vi "autonomous hard code.vi"   [LabVIEW 2012]
uses:
  <vilib>/Platform/TimedLoop/XDataNode/timing_clust.ctl
  <vilib>/Platform/TimedLoop/XDataNode/nitl_modes.ctl
  <vilib>/Platform/TimedLoop/XDataNode/wakeup.ctl
  <vilib>/Rock Robotics/WPI/RobotDrive/WPI_RobotDriveArcadeDrive_Standard(NoSaturation).vi
  <vilib>/Rock Robotics/WPI/RobotDrive/WPI_RobotDriveGetSetRefNum.vi
  <vilib>/platform/TimedLoop/XDataNode/XDataNode.xnode
  <vilib>/Platform/TimedLoop/XDataNode/XDNodeRunTimeDep.lvlib
types:
  T1 = typedef "XDNodeRunTimeDep.lvlib/timing_clust.ctl" = cluster{"Expected End [f-1]":u64, "Actual End [f-1]":u64, "Finished Late? [f-1]":bool, "Expected End [i-1]":u64, "Actual End [i-1]":u64, "Finished Late? [i-1]":bool, "Expected Start [i]":u64, "Actual Start [i]":u64, "Expected Start [f]":u64, "Actual Start [f]":u64, "Source Name":string, "Structure Name":string, "Period":i64, "Deadline":i64, "Offset":i64, "Start":i64, "Priority":i32, "Timeout":i32, "Mode":T2, "Wakeup Reason":T3, "Error":errorcluster, "Source Type":string, "Secondary Source Type":string, "Global End Time":u64, "Global Start Time":u64, "Frame Duration":u64, "Iteration Duration":u64, "Assigned CPU":i32, "I/O Scan Engine Mode":u32}
  T2 = typedef "XDNodeRunTimeDep.lvlib/nitl_modes.ctl" = enum32{"No Change", "Process missed periods, maintain original phase", "Discard missed periods, maintain original phase", "Process missed periods, ignore original phase", "Discard missed periods, ignore original phase"}
  T3 = typedef "XDNodeRunTimeDep.lvlib/wakeup.ctl" = enum32{"Normal", "Aborted", "Asynchronous wakeup", "Timing source error", "Timed loop error", "Timeout"}
  T4 = typedef "WPI_RobotDriveDevRef.ctl" = cluster{"DevStatus":errorcluster, "Motors[]":T5[], "Square Inputs":bool, "Max Output":dbl, "Isochronous":bool}
  T5 = typedef "WPI_MotorControlDeviceRef.ctl" = cluster{"DeviceStatus":errorcluster, "Type":enum16{"PWM", "CAN"}, "PWM":cluster{"Digital Module":T6, "PWM Channel":T7, "DeadBand":T8}, "CAN":cluster{"Device Number":u8, "Control Mode":T9, "Semaphore":T10, "Max Vout":dbl}, "Invert":bool, "TransformRef":T11, "InvTransformRef":T11}
  T6 = typedef "FPGA_TypedefDigitalModule.ctl" = enum16{"Digital Module 1", "Digital Module 2"}
  T7 = typedef "FPGA_DIOPWMChannel.ctl" = enum8{"PWM 1", "PWM 2", "PWM 3", "PWM 4", "PWM 5", "PWM 6", "PWM 7", "PWM 8", "PWM 9", "PWM 10", "Invalid"}
  T8 = typedef "WPI_PWMDeadband.ctl" = cluster{"Name":string, "maxPositivePwm":i32, "minPositivePwm":i32, "centerPwm":i32, "maxNegativePwm":i32, "minNegativePwm":i32, "angularRange":u16}
  T9 = typedef "WPI_CANJaguar_ControlMode.ctl" = enum8{"Percent VBus", "Current", "Speed", "Position", "Voltage"}
  T10 = typedef "Semaphore RefNum" = refnum<k1>
  T11 = typedef "WPI_PWMTransform_ConPane.ctl" = refnum<vi>
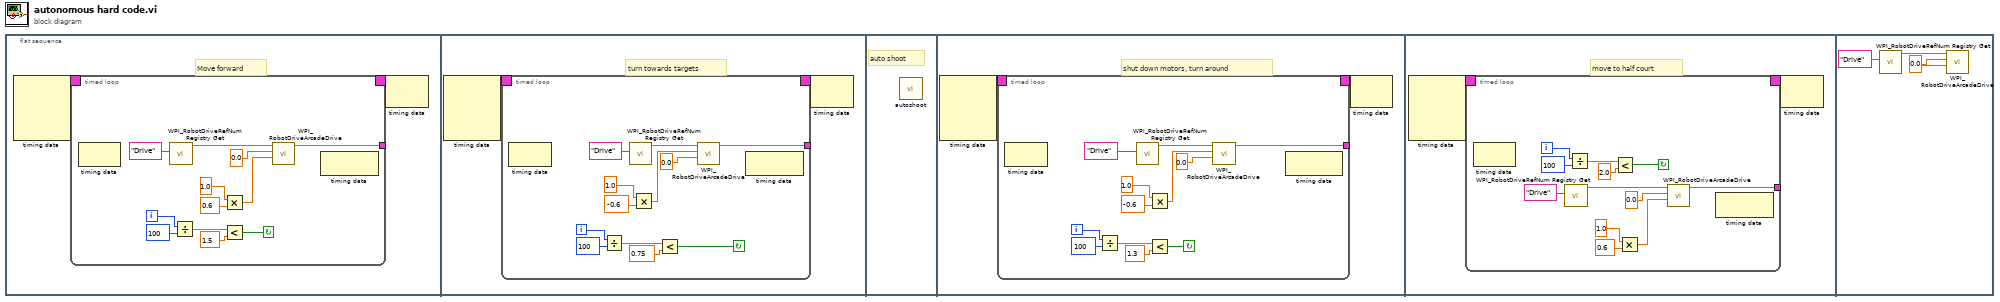
[diagram p0: block diagram]
diagram:
  n1 = flat-sequence {
    frame #0 {
      # "Move forward"
      n2 = node-c288() -> (w2:T1)  [unwired: 4 in]
      n3 = timed-loop {
        timing: w2 -> [_]
        timing-out: [_] -> w1
        tunnel: [w8] -> _
        i -> [w7]
        stop <- w14 continue-if-true
        n4 = node-c288() -> ()  [unwired: 1 in, 1 out]
        n5 = call <vilib>:"WPI_RobotDriveRefNum Registry Get.vi"("refnum name"="Drive") -> ("RobotDriveDevRef"=w10:T4)  [unwired: 9 in, 1 out]
        n6 = Divide(x=w7, y=100) -> (x/y=w12:dbl)
        n7 = Multiply(x=1.0, y=0.6) -> (x*y=w3:dbl)
        n8 = Less?(x=w12, y=1.5) -> (x < y?=w14:bool)
        n9 = call-poly <vilib>:"WPI_RobotDriveArcadeDrive.vi"("Y axis value"=w3, "X axis value"=0.0 ("Y axis value"), "RobotDriveDevRef"=w10) -> ("RobotDriveDevRef"=w8:T4)  [unwired: 6 in, 2 out]
        n10 = node-c288() -> ()  [unwired: 1 in, 1 out]
      }
      n11 = node-c288(w1) -> ()  [unwired: 1 out]
    }
    frame #1 {
      # "turn towards targets"
      n12 = node-c288() -> (w20:T1)  [unwired: 4 in]
      n13 = timed-loop {
        timing: w20 -> [_]
        timing-out: [_] -> w19
        tunnel: [w24] -> _
        i -> [w23]
        stop <- w32 continue-if-true
        n14 = node-c288() -> ()  [unwired: 1 in, 1 out]
        n15 = Divide(x=w23, y=100) -> (x/y=w30:dbl)
        n16 = call <vilib>:"WPI_RobotDriveRefNum Registry Get.vi"("refnum name"="Drive") -> ("RobotDriveDevRef"=w28:T4)  [unwired: 9 in, 1 out]
        n17 = Multiply(x=1.0, y=-0.6) -> (x*y=w27:dbl)
        n18 = Less?(x=w30, y=0.75) -> (x < y?=w32:bool)
        n19 = call-poly <vilib>:"WPI_RobotDriveArcadeDrive.vi"("Y axis value"=0.0, "X axis value"=w27, "RobotDriveDevRef"=w28) -> ("RobotDriveDevRef"=w24:T4)  [unwired: 6 in, 2 out]
        n20 = node-c288() -> ()  [unwired: 1 in, 1 out]
      }
      n21 = node-c288(w19) -> ()  [unwired: 1 out]
    }
    frame #2 {
      # "auto shoot"
      n22 = call "autoshoot.vi"() -> ()  [unwired: 12 in]
    }
    frame #3 {
      # "shut down motors, turn around"
      n23 = node-c288() -> (w38:T1)  [unwired: 4 in]
      n24 = timed-loop {
        timing: w38 -> [_]
        timing-out: [_] -> w37
        tunnel: [w42] -> _
        i -> [w41]
        stop <- w50 continue-if-true
        n25 = node-c288() -> ()  [unwired: 1 in, 1 out]
        n26 = Divide(x=w41, y=100) -> (x/y=w48:dbl)
        n27 = call <vilib>:"WPI_RobotDriveRefNum Registry Get.vi"("refnum name"="Drive") -> ("RobotDriveDevRef"=w46:T4)  [unwired: 9 in, 1 out]
        n28 = Multiply(x=1.0, y=-0.6) -> (x*y=w45:dbl)
        n29 = Less?(x=w48, y=1.3) -> (x < y?=w50:bool)
        n30 = call-poly <vilib>:"WPI_RobotDriveArcadeDrive.vi"("Y axis value"=0.0, "X axis value"=w45, "RobotDriveDevRef"=w46) -> ("RobotDriveDevRef"=w42:T4)  [unwired: 6 in, 2 out]
        n31 = node-c288() -> ()  [unwired: 1 in, 1 out]
      }
      n32 = node-c288(w37) -> ()  [unwired: 1 out]
    }
    frame #4 {
      # "move to half court"
      n33 = node-c288() -> (w56:T1)  [unwired: 4 in]
      n34 = timed-loop {
        timing: w56 -> [_]
        timing-out: [_] -> w55
        tunnel: [w62] -> _
        i -> [w61]
        stop <- w68 continue-if-true
        n35 = node-c288() -> ()  [unwired: 1 in, 1 out]
        n36 = call <vilib>:"WPI_RobotDriveRefNum Registry Get.vi"("refnum name"="Drive") -> ("RobotDriveDevRef"=w64:T4)  [unwired: 9 in, 1 out]
        n37 = Divide(x=w61, y=100) -> (x/y=w66:dbl)
        n38 = Less?(x=w66, y=2.0) -> (x < y?=w68:bool)
        n39 = Multiply(x=1.0, y=0.6) -> (x*y=w57:dbl)
        n40 = call-poly <vilib>:"WPI_RobotDriveArcadeDrive.vi"("Y axis value"=w57, "X axis value"=0.0 ("Y axis value"), "RobotDriveDevRef"=w64) -> ("RobotDriveDevRef"=w62:T4)  [unwired: 6 in, 2 out]
        n41 = node-c288() -> ()  [unwired: 1 in, 1 out]
      }
      n42 = node-c288(w55) -> ()  [unwired: 1 out]
    }
    frame #5 {
      w73 = 0.0 ("X axis value")
      n43 = call <vilib>:"WPI_RobotDriveRefNum Registry Get.vi"("refnum name"="Drive") -> ("RobotDriveDevRef"=w75:T4)  [unwired: 9 in, 1 out]
      n44 = call-poly <vilib>:"WPI_RobotDriveArcadeDrive.vi"("Y axis value"=w73, "X axis value"=w73, "RobotDriveDevRef"=w75) -> ()  [unwired: 6 in, 3 out]
    }
  }
